vi "Create PDFWriter.vi"(0 "PDF Report IN":refnum<class "PDF Report Class.lvclass">, 2 "At the opening":T1={"Page"=0, "Show Bookmarks"=TRUE} {"Page" items=["Single Page - Fit Page"=1, "Single Page - Fit Width"=0]}, 11 "error in (no error)":errorcluster) -> (4 "PDF Report OUT":refnum<class "PDF Report Class.lvclass">, 15 "error out":errorcluster)   [LabVIEW 2019, in "Exaprom PDF.lvlib"]
doc: "Version 2.0\nDeveloped by Jean-Marc Simard\nCopyright © 2013, Exaprom Inc.\nAll rights reserved.\nLicense: BSD\n\nWith iTextSharp 4.1.6 (http://itextsharp.sourceforge.net)\nunder Mozilla Public License Version 1.1\n(http://www.mozilla.org/MPL/MPL-1.1.html)"
uses:
  LV Class/PDF Report Class/PDF Report Class.lvclass
  Controls/Initialization Controls/At the opening.ctl
  C:/work/niobrara_lv/labview pdf writer fixing/DLL/itextsharp.dll
  DLL/itextsharp.dll
  Exaprom PDF.lvlib
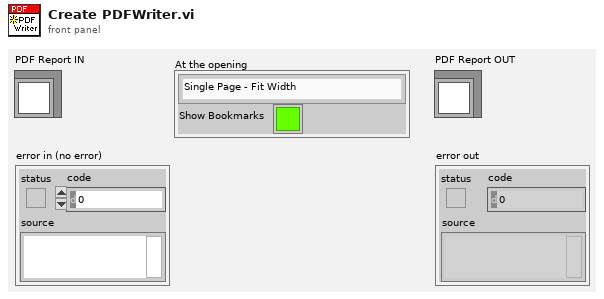
[diagram p1: front panel]
types:
  T1 = typedef "Exaprom PDF.lvlib/At the opening.ctl" = cluster{"Page":u16, "Show Bookmarks":bool}
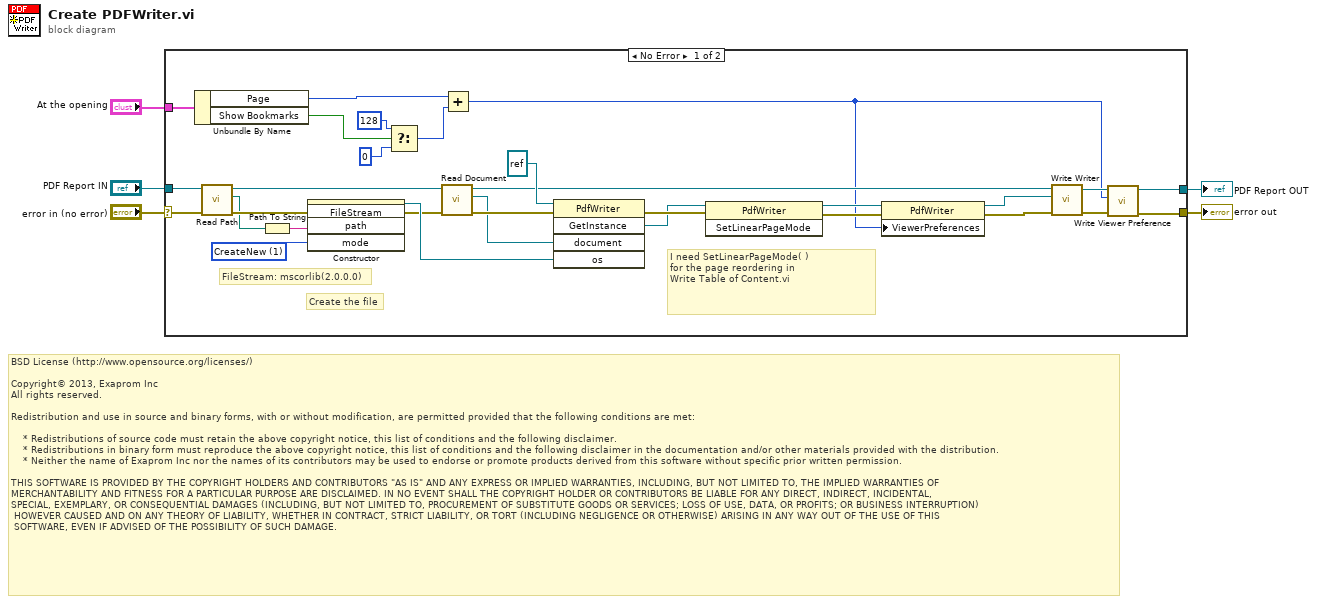
[diagram p0: block diagram]
diagram:
  # "BSD License (http://www.opensource.org/licenses/)\n\nCopyright© 2013, Exaprom Inc\nAll rights reserved.\n\nRedistribution and use in source and binary forms, with or without modification, are permitted provided that the following conditions are met:\n\n    * Redistributions of source code must retain the above copyright notice, this list of conditions and the following disclaimer.\n    * Redistributions in binary form must reproduce the above copyright notice, this list of conditions and the following disclaimer in the documentation and/or other materials provided with the distribution.\n    * Neither the name of Exaprom Inc nor the names of its contributors may be used to endorse or promote products derived from this software without specific prior written permission.\n\nTHIS SOFTWARE IS PROVIDED BY THE COPYRIGHT HOLDERS AND CONTRIBUTORS \"AS IS\" AND ANY EXPRESS OR IMPLIED WARRANTIES, INCLUDING, BUT NOT LIMITED TO, THE IMPLIED WARRANTIES OF \nMERCHANTABILITY AND FITNESS FOR A PARTICULAR PURPOSE ARE DISCLAIMED. IN NO EVENT SHALL THE COPYRIGHT HOLDER OR CONTRIBUTORS BE LIABLE FOR ANY DIRECT, INDIRECT, INCIDENTAL,\nSPECIAL, EXEMPLARY, OR CONSEQUENTIAL DAMAGES (INCLUDING, BUT NOT LIMITED TO, PROCUREMENT OF SUBSTITUTE GOODS OR SERVICES; LOSS OF USE, DATA, OR PROFITS; OR BUSINESS INTERRUPTION)\n HOWEVER CAUSED AND ON ANY THEORY OF LIABILITY, WHETHER IN CONTRACT, STRICT LIABILITY, OR TORT (INCLUDING NEGLIGENCE OR OTHERWISE) ARISING IN ANY WAY OUT OF THE USE OF THIS\n SOFTWARE, EVEN IF ADVISED OF THE POSSIBILITY OF SUCH DAMAGE."
  n1 = case shown="No Error" "error in (no error)" {
    selector: "error in (no error)" -> [w30 w37]
    tunnel: "PDF Report IN" -> [w29 w36]
    tunnel: [w9 w36] -> w4
    tunnel: [w7 w37] -> w3
    tunnel: "At the opening" -> [w15 _]
    frame No Error {
      w33 = 1 items=["CreateNew"=1, "Create"=2, "Open"=3, "OpenOrCreate"=4, "Truncate"=5, "Append"=6] ("mode")
      # "I need SetLinearPageMode( )\nfor the page reordering in \nWrite Table of Content.vi"
      # "Create the file"
      # "FileStream: mscorlib(2.0.0.0)"
      n2 = Unbundle By Name(w15) -> ("Page"=w12:u16, "Show Bookmarks"=w14:bool)
      n3 = call-dynamic "Read Path.vi"("error in (no error)"=w30, "PDF Report Class in"=w29) -> ("error out"=w31:errorcluster, "Path"=w28:path, "PDF Report Class out"=w26:refnum<class "PDF Report Class.lvclass">)  [unwired: 7 in]
      n4 = Path To String(path=w28) -> (string=w34:string)
      n5 = constructor class="FileStream" ("Constructor Node")(error in=w31, "path"=w34, "mode"=w33) -> (reference out=w32:refnum<k24>, error out=w25:errorcluster)  [unwired: 2 in, 3 out]
      n6 = Select(t=128 ("ViewerPreferences"), s=w14, f=0) -> (s? t:f=w11:i32)
      n7 = call-dynamic "Read Document.vi"("error in (no error)"=w25, "PDF Report Class in"=w26) -> ("error out"=w24:errorcluster, "Document"=w23:refnum<k24>, "PDF Report Class out"=w27:refnum<class "PDF Report Class.lvclass">)  [unwired: 7 in]
      n8 = Add(x=w12, y=w11) -> (x+y=w6:i32)
      n9 = invoke class="PdfWriter" method="GetInstance"(reference=refnum<k24> refnum, error in=w24, "document"=w23, "os"=w32) -> (error out=w21:errorcluster, "GetInstance"=w20:refnum<k24>)  [unwired: 1 in, 3 out]
      n10 = invoke class="PdfWriter" method="SetLinearPageMode"(reference=w20, error in=w21) -> (reference out=w17:refnum<k24>, error out=w19:errorcluster)  [unwired: 1 in, 1 out]
      n11 = property class="PdfWriter"(reference=w17, error in=w19, "ViewerPreferences"=w6) -> (reference out=w16:refnum<k24>, error out=w18:errorcluster)
      n12 = call-dynamic "Write Writer.vi"("error in (no error)"=w18, "Writer"=w16, "PDF Report Class in"=w27) -> ("error out"=w8:errorcluster, "PDF Report Class out"=w22:refnum<class "PDF Report Class.lvclass">)  [unwired: 7 in]
      n13 = call-dynamic "Write Viewer Preference.vi"("error in (no error)"=w8, "Viewer Preference"=w6, "PDF Report Class in"=w22) -> ("error out"=w7:errorcluster, "PDF Report Class out"=w9:refnum<class "PDF Report Class.lvclass">)  [unwired: 7 in]
    }
    frame Error {
    }
  }
  "PDF Report OUT" <- w4
  "error out" <- w3
